vi "Keithley 27XX Connect and Read Buffer.vi"() -> ()   [LabVIEW 2020]
doc: "This Example can be used to connect to the instrument and download the data buffer after a measurement has already occured."
uses:
  <instrlib>/Keithley 27XX/Public/Data/Read Data Buffer.vi
  <instrlib>/Keithley 27XX/Keithley 27XX.lvlib
panel:
  in  "Serial Configuration":T1={"Baud Rate (9600)"=9600, "Flow Control (1: XON/XOFF)"=1, "Termination Char (0:CR)"=0} {"Termination Char (0:CR)" items=["CR", "LF"]; "Flow Control (1: XON/XOFF)" items=["None", "XON/XOFF", "RTS/CTS (2701 Only)", "XON/XOFF & RTS/CTS (2701 Only)"]; "Baud Rate (9600)" items=["300"=300, "600"=600, "1200"=1200, "2400"=2400, "4800"=4800, "9600"=9600, "19.2k"=19200, "38.4k (2701 Only)"=38400, "57.6k (2701 Only)"=57600, "115.2k (2701 Only)"=115200]}
  in  "Timeout (30000 milliseconds)":u32=30000
  out "Measurement Data":dbl[](array[numeric])
  in  "VISA resource name":refnum<visa-resource-name>
  # "© 2005 National Instruments Corporation.  ALL RIGHTS RESERVED."
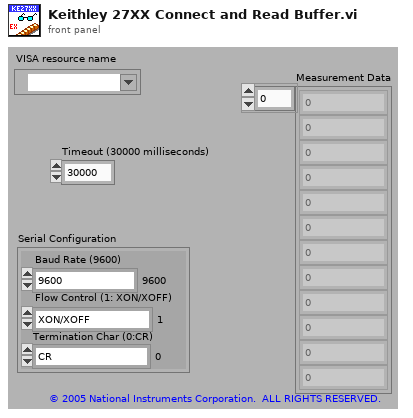
[diagram p1: front panel]
types:
  T1 = cluster{"Baud Rate (9600)":u32, "Flow Control (1: XON/XOFF)":u16, "Termination Char (0:CR)":u16}
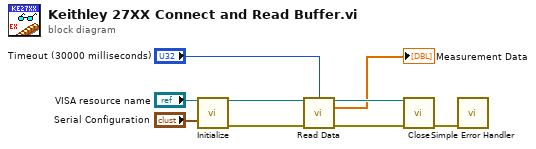
[diagram p0: block diagram]
diagram:
  n1 = call <instrlib>:"Initialize.vi"("VISA resource name"="VISA resource name", "Serial Configuration"="Serial Configuration") -> ("VISA resource name out"=w9:refnum<visa-resource-name>, "error out"=w8:errorcluster)  [unwired: 12 in]
  n2 = call-poly <instrlib>:"Read Data.vi"("VISA resource name"=w9, "Timeout (30000 milliseconds)"="Timeout (30000 milliseconds)", "error in (no error)"=w8) -> ("VISA resource name out"=w6:refnum<visa-resource-name>, "Measurement Data"=→"Measurement Data":dbl[], "error out"=w7:errorcluster)  [unwired: 7 in, 3 out]
  n3 = call <instrlib>:"Close.vi"("VISA resource name"=w6, "error in (no error)"=w7) -> ("error out"=w5:errorcluster)  [unwired: 13 in]
  n4 = call <vilib>:"Simple Error Handler.vi"("error in (no error)"=w5) -> ()  [unwired: 4 in, 5 out]
